vi "fgt set all Valves.vi"(8 "error in (no error)":errorcluster, 9 "position":i32, 10 "moduleIndex":u32, 11 "controllerIndex":u32) -> (0 "error out":errorcluster)   [LabVIEW 2020, in "fgt_SDK.lvlib"]
doc: "Set power ON or OFF on a controller (such as Link, MFCS, Flowboard).\nNot all controllers support this functionality."
uses:
  fgt_SDK.lvlib
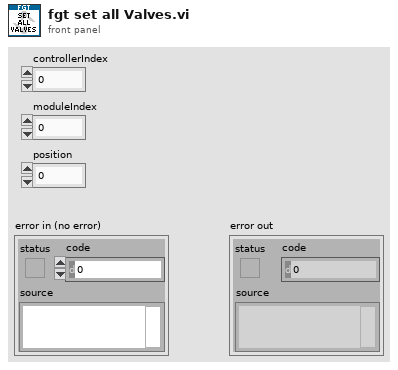
[diagram p1: front panel]
types:
  T1 = typedef "fgt_SDK.lvlib/fgt_STATUS_INFO.ctl" = cluster{"InstrType":T2, "instrSN":u16, "errorCode":u8, "infoCode":u8, "detail":string}
  T2 = typedef "fgt_SDK.lvlib/fgt_INSTRUMENT_TYPE.ctl" = enum32{"None", "MFCS", "MFCS_EZ", "FRP", "LineUP", "IPS"}
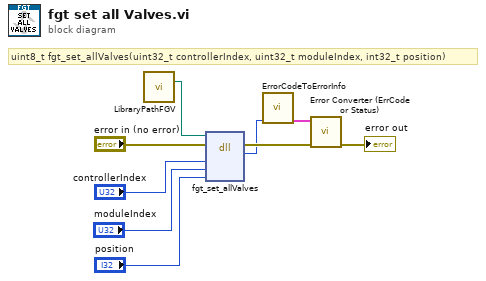
[diagram p0: block diagram]
diagram:
  # "uint8_t fgt_set_allValves(uint32_t controllerIndex, uint32_t moduleIndex, int32_t position)"
  n1 = call "LibraryPathFGV.vi"() -> ("Path Out"=w1:path)  [unwired: 14 in, 1 out]
  n2 = dll-call lib="C:/Workspace/fgt-SDK/LabVIEW/dlls/fgt_SDK_*.*" fn="fgt_set_allValves"(path in=w1, error in="error in (no error)", "controllerIndex"="controllerIndex", "moduleIndex"="moduleIndex", "position"="position") -> (error out=w7:errorcluster, "return type"=w5:u8)  [unwired: 4 in, 1 out]
  n3 = call "ErrorCodeToErrorInfo.vi"("return type"=w5) -> ("StatusInfo"=w4:T1)  [unwired: 10 in]
  n4 = call "Error Converter (ErrCode or Status).vi"("error in (no error)"=w7, "StatusInfo"=w4) -> ("error out"=→"error out":errorcluster)  [unwired: 9 in]
